vi "use gyro to drive straight.vi"(8 "OG Gyro":dbl, 9 "RightDriveIn":dbl, 10 "LeftDriveIn":dbl) -> (1 "RightDriveOut":dbl, 2 "LeftDriveOut":dbl)   [LabVIEW 2017]
uses:
  Robot Global Data.vi
panel:
  in  "Gyro kP":dbl
  # "need to tune otherwise it does nothing"
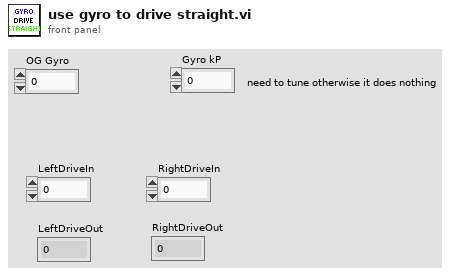
[diagram p1: front panel]
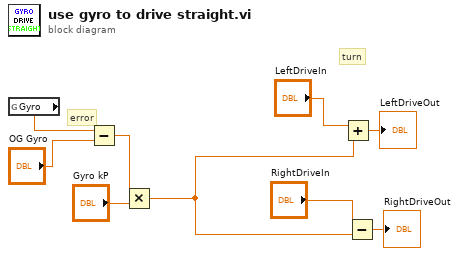
[diagram p0: block diagram]
diagram:
  # "turn"
  # "error"
  n1 = global read "Robot Global Data.vi" "Gyro"() -> (w1:dbl)
  n2 = Subtract(x=w1, y="OG Gyro") -> (x-y=w9:dbl)
  n3 = Multiply(x=w9, y="Gyro kP") -> (x*y=w4:dbl)
  n4 = Add(x="LeftDriveIn", y=w4) -> (x+y=→"LeftDriveOut":dbl)
  n5 = Subtract(x="RightDriveIn", y=w4) -> (x-y=→"RightDriveOut":dbl)
